vi "DataProcessorDEM.vi"(0 "DATA in":refnum<queue>, 3 "FPGA in":refnum<queue>) -> ()   [LabVIEW 2019, in "FPGA.lvlib"]
uses:
  FPGA.lvlib
  FPGA.ctl
  ResultSweep.vi
panel:
  out "theta 2":dbl
  out "r 2":dbl
  out "theta":dbl
  out "r":dbl
  out "Waveform Graph 2":dbl[](graph)
  out "Waveform Graph":dbl[](graph)
  out "Module":cluster{dbl[], dbl[]}(graph)
  out "Phase":cluster{dbl[], dbl[]}(graph)
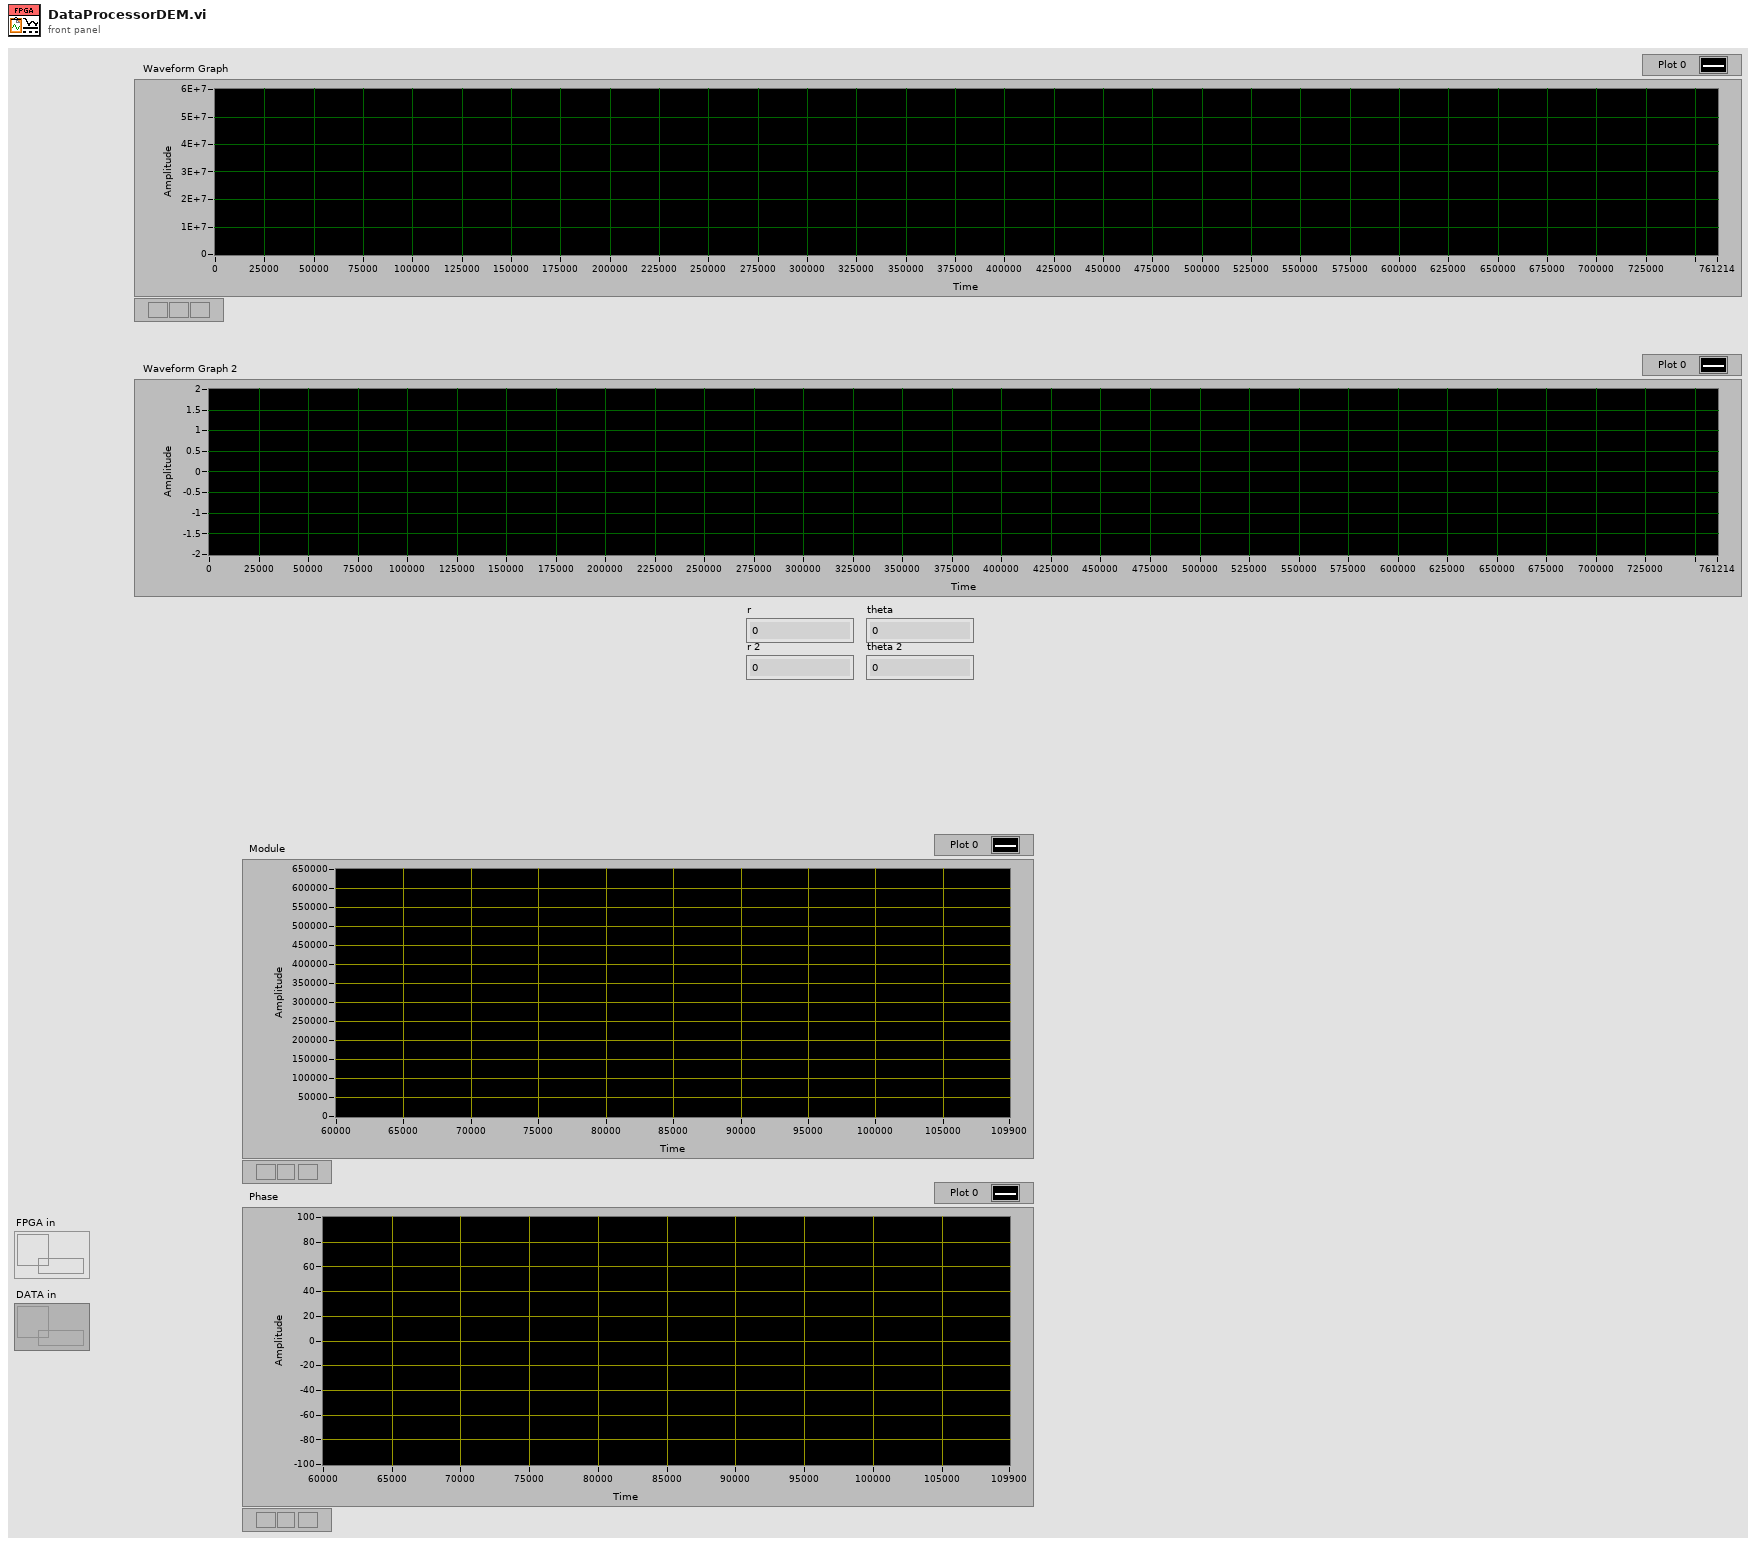
[diagram p1: front panel]
types:
  T1 = typedef "FPGA.lvlib/FPGA.ctl" = cluster{"Start freq. [Hz]":dbl, "Sweep duration [s]":dbl, "Freq. step [Hz]":dbl, "DAC Sample Rate":dbl, "ADC Sample Rate":dbl, "CMD port":u16, "DFAST port":u16, "CMD ID":refnum<k16>, "DFAST ID":refnum<k16>, "CMD error out":errorcluster, "FPGA IP":string, "DFAST error out ":errorcluster, "Stop freq. [Hz]":dbl, "Discrete sweep":bool, "Initial NCO":u32, "Difference NCO":i32, "step NCO":i64, "Final NCO":u32, "clocks for step":u32, "demodulation":bool, "NCO Phase Precision":u32, "NCO Sample Rate":dbl, "Time for step [s]":dbl, "NCO freq. resolution":dbl, "Sweep speed [Hz/s]":dbl, "Connected":bool, "Slew Rate [V/us]":dbl, "Parameters_ok":bool, "Amplitude [mVpp]":dbl, "Scale Factor":fxp<+,16,0>, "Acquiring":bool, "DAC-ADC Latency":u16, "Digital Gain":i32, "Number of steps":i32, "Averaging preferred":bool, "Filter Order":u32, "Settling":enum16{"99%", "99,9%"}}
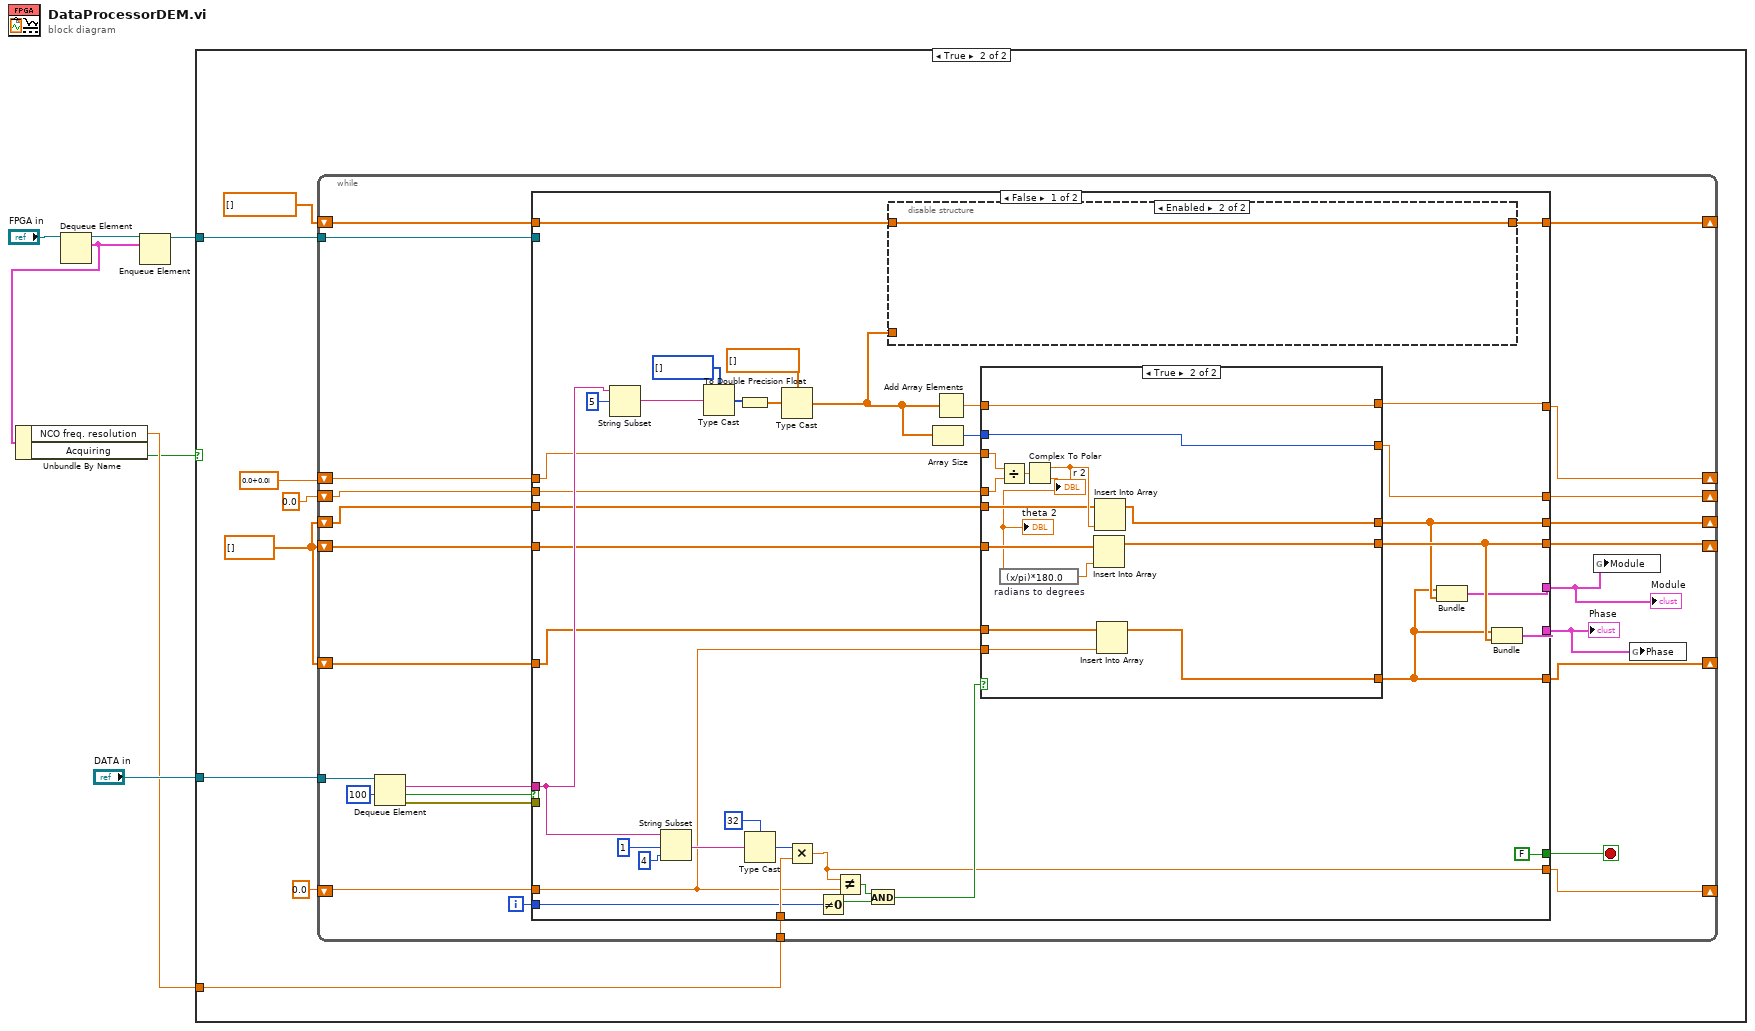
[diagram p0: block diagram]
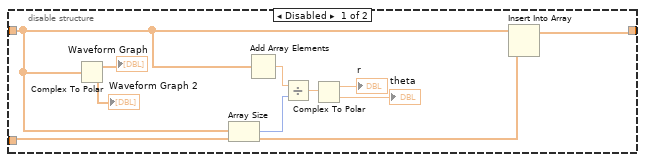
[diagram p3: hidden frame]
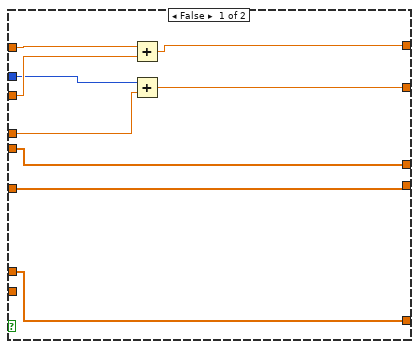
[diagram p4: hidden frame]
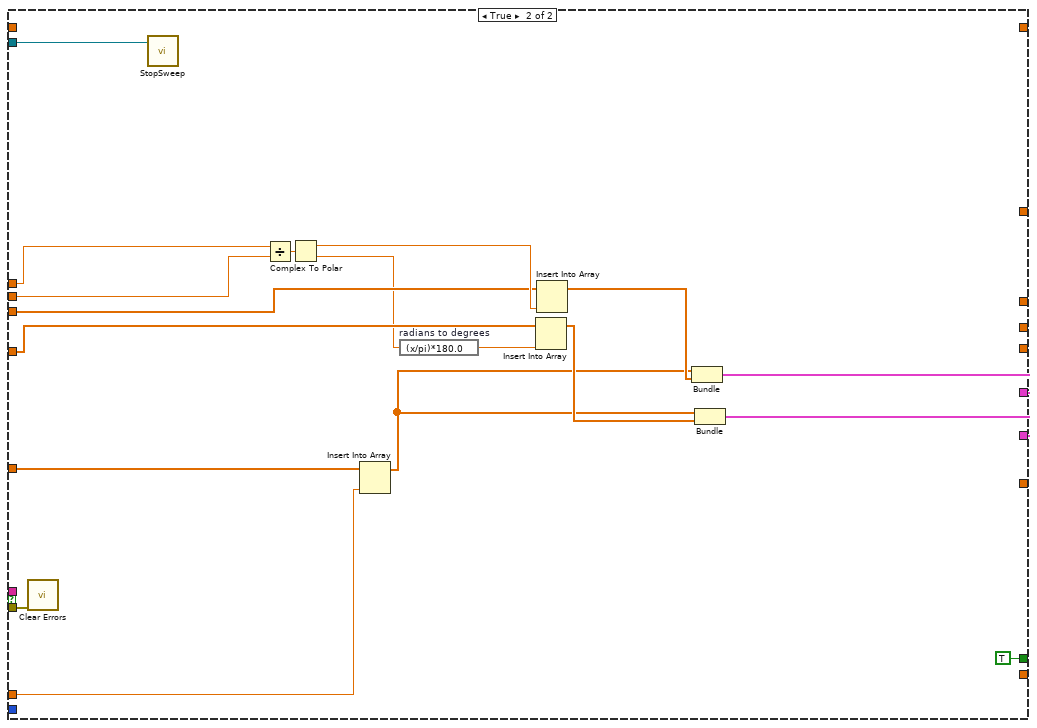
[diagram p5: hidden frame]
diagram:
  n1 = Dequeue Element(queue="FPGA in") -> (queue out=w3:refnum<queue>, element=w2:T1)  [unwired: 2 in, 2 out]
  n2 = Unbundle By Name(w2) -> ("NCO freq. resolution"=w5:dbl, "Acquiring"=w4:bool)
  n3 = Enqueue Element(queue=w3, element=w2) -> (queue out=w1:refnum<queue>)  [unwired: 2 in, 2 out]
  n4 = case shown="True" w4 {
    tunnel: w5 -> [_ w14]
    tunnel: "DATA in" -> [_ w15]
    tunnel: w1 -> [_ w12]
    frame False {
    }
    frame True {
      w9 = dbl[] []
      n5 = while {
        tunnel: w15 -> [w39]
        shift-right: [w33] -> _
        shift-left: 0.0 ("length (rest)") -> [w34]
        tunnel: w14 -> [w36]
        shift-right: [w30] -> _
        shift-left: cdb 0.0+0.0i -> [w35]
        shift-right: [w31] -> _
        shift-left: 0.0 -> [w32]
        shift-right: [w28] -> _
        shift-left: w9 -> [w29]
        shift-right: [w25] -> _
        shift-left: w9 -> [w26]
        tunnel: w12 -> [w24]
        shift-right: [w22] -> _
        shift-left: w9 -> [w23]
        shift-right: [w17] -> _
        shift-left: cdb[] [] -> [w18]
        i -> [w27]
        stop <- w16 stop-if-true
        n6 = Dequeue Element(queue=w39, timeout in ms (-1)=100) -> (element=w38:string, timed out?=w21:bool, error out=w37:errorcluster)  [unwired: 1 in, 1 out]
        n7 = case shown="False" w21 {
          tunnel: w38 -> [w75 _]
          tunnel: w37 -> [_ w130]
          tunnel: w36 -> [w72 _]
          tunnel: w35 -> [w71 w117]
          tunnel: w34 -> [w61 w128]
          tunnel: [w62 _] -> w33
          tunnel: w32 -> [w70 w116]
          tunnel: [w52 _] -> w31
          tunnel: [w51 _] -> w30
          tunnel: w29 -> [w69 w118]
          tunnel: [w49 _] -> w28
          tunnel: w27 -> [w67 _]
          tunnel: w26 -> [w63 w129]
          tunnel: [w45 _] -> w25
          tunnel: w24 -> [_ w127]
          tunnel: w23 -> [w50 w119]
          tunnel: [w47 _] -> w22
          tunnel: [w46 w122] -> w20
          tunnel: [w48 w121] -> w19
          tunnel: w18 -> [w44 _]
          tunnel: [w42 _] -> w17
          tunnel: [FALSE TRUE] -> w16
          frame False {
            n8 = String Subset(string=w75, offset (0)=5) -> (substring=w55:string)  [unwired: 1 in]
            n9 = String Subset(string=w75, offset (0)=1, length (rest)=4 ("length (rest)")) -> (substring=w74:string)
            n10 = Type Cast(type=i32[] [], x=w55) -> (*(type *) &x=w59:i32[])
            n11 = To Double Precision Float(number=w59) -> (double precision float=w58:dbl[])
            n12 = Type Cast(type=u32 32 ("length (rest)"), x=w74) -> (*(type *) &x=w68:u32)
            n13 = Type Cast(type=cdb[] [], x=w58) -> (*(type *) &x=w43:cdb[])
            n14 = Multiply(x=w68, y=w72) -> (x*y=w62:dbl)
            n15 = Not Equal To 0?(x=w67) -> (x != 0?=w65:bool)
            n16 = Not Equal?(x=w62, y=w61) -> (x != y?=w66:bool)
            n17 = And(x=w66, y=w65) -> (x .and. y?=w64:bool)
            n18 = disable-structure shown="Enabled" {
              disable-tunnel: w44 -> [w78 w88]
              disable-tunnel: w43 -> [w87 _]
              disable-tunnel: [w79 w88] -> w42
              frame Disabled {
                n19 = Complex To Polar(r * e^(i*theta)=w78) -> (r=→"Waveform Graph":dbl[], theta=→"Waveform Graph 2":dbl[])
                n20 = Array Size(array=w78) -> (size(s)=w83:i32)
                n21 = Add Array Elements(numeric array=w78) -> (sum=w84:cdb)
                n22 = Divide(x=w84, y=w83) -> (x/y=w82:cdb)
                n23 = Complex To Polar(r * e^(i*theta)=w82) -> (r=→"r":dbl, theta=→"theta":dbl)
                n24 = Insert Into Array(array=w78, new element=w87) -> (w79:cdb[])  [unwired: 1 in]
              }
              frame Enabled {
              }
            }
            n25 = Array Size(array=w43) -> (size(s)=w53:i32)
            n26 = Add Array Elements(numeric array=w43) -> (sum=w54:cdb)
            n27 = case shown="True" w64 {
              tunnel: [w93 w112] -> w51
              tunnel: w54 -> [w95 w112]
              tunnel: w71 -> [w94 w107]
              tunnel: w70 -> [w91 w106]
              tunnel: [w90 w108] -> w52
              tunnel: w69 -> [w97 w111]
              tunnel: [w97 w101] -> w49
              tunnel: w63 -> [w96 w110]
              tunnel: [w96 w100] -> w45
              tunnel: w61 -> [_ w109]
              tunnel: w53 -> [w92 w108]
              tunnel: w50 -> [w89 w103]
              tunnel: [w89 w102] -> w47
              frame False {
                n28 = Add(x=w95, y=w94) -> (x+y=w93:cdb)
                n29 = Add(x=w92, y=w91) -> (x+y=w90:dbl)
              }
              frame True {
                n30 = Divide(x=w107, y=w106) -> (x/y=w105:cdb)
                n31 = Complex To Polar(r * e^(i*theta)=w105) -> (r=w104:dbl, theta=w98:dbl)
                "r 2" <- w104
                "theta 2" <- w98
                n32 = expression code="(x/pi)*180.0" "radians to degrees"(w98) -> (w99:dbl)
                n33 = Insert Into Array(array=w111, new element=w99) -> (w101:dbl[])  [unwired: 1 in]
                n34 = Insert Into Array(array=w103, new element=w104) -> (w102:dbl[])  [unwired: 1 in]
                n35 = Insert Into Array(array=w110, new element=w109) -> (w100:dbl[])  [unwired: 1 in]
              }
            }
            n36 = Bundle(w45, w47) -> (w46:cluster{dbl[], dbl[]})  [unwired: 1 in]
            n37 = Bundle(w45, w49) -> (w48:cluster{dbl[], dbl[]})  [unwired: 1 in]
          }
          frame True {
            n38 = call <vilib>:"Clear Errors.vi"("error in (no error)"=w130) -> ()  [unwired: 5 in, 2 out]
            n39 = call "StopSweep.vi"("FPGA in"=w127) -> ()  [unwired: 10 in, 1 out]
            n40 = Divide(x=w117, y=w116) -> (x/y=w126:cdb)
            n41 = Complex To Polar(r * e^(i*theta)=w126) -> (r=w125:dbl, theta=w114:dbl)
            n42 = Insert Into Array(array=w129, new element=w128) -> (w120:dbl[])  [unwired: 1 in]
            n43 = expression code="(x/pi)*180.0" "radians to degrees"(w114) -> (w115:dbl)
            n44 = Insert Into Array(array=w118, new element=w115) -> (w123:dbl[])  [unwired: 1 in]
            n45 = Insert Into Array(array=w119, new element=w125) -> (w124:dbl[])  [unwired: 1 in]
            n46 = Bundle(w120, w124) -> (w122:cluster{dbl[], dbl[]})  [unwired: 1 in]
            n47 = Bundle(w120, w123) -> (w121:cluster{dbl[], dbl[]})  [unwired: 1 in]
          }
        }
        "Module" <- w20
        "Phase" <- w19
        n48 = global write "ResultSweep.vi" "Module"(w20) -> ()
        n49 = global write "ResultSweep.vi" "Phase"(w19) -> ()
      }
    }
  }
